vi "Goal Vision Align.vi"(10 "reinitialize? (F)":bool, 11 "Goal Vision Packet":T1) -> (1 "Heading Target":dbl, 2 "Aligned?":bool, 3 "Turn Power":dbl)   [LabVIEW 2015]
uses:
  Common Code/Goal Vision Packet.ctl
  Robot Global Data.vi
  <vilib>/addons/control/pid/pid.llb/PID (DBL).vi
  <vilib>/addons/control/pid/NI_PID_pid.lvlib
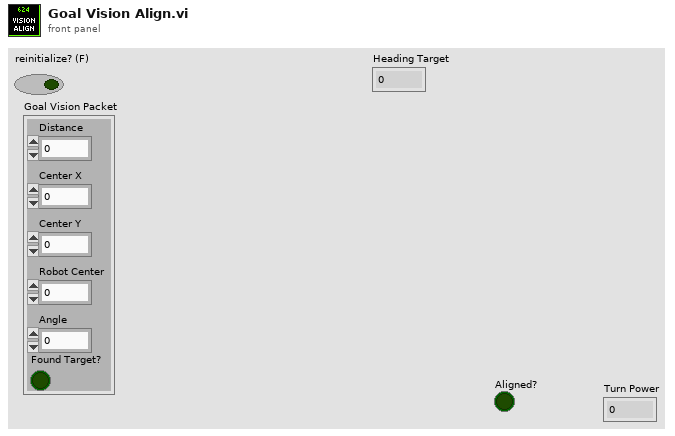
[diagram p1: front panel]
types:
  T1 = typedef "Goal Vision Packet.ctl" = cluster{"Distance":dbl, "Center X":dbl, "Center Y":dbl, "Found Target?":bool, "Robot Center":dbl, "Angle":dbl}
  T2 = typedef "Dashboard Control Data.ctl" = cluster{"Shooter Presets":T3, "Encoder Control":T5, "Steer PID output":cluster{"output high":dbl, "output low":dbl}, " Steer PID gains":cluster{"proportional gain (Kc)":dbl, "integral time (Ti, min)":dbl, "derivative time (Td, min)":dbl}, "Drivetrain Settings":T6, "Vision Packet":T1, "Dashboard Drivetrain Command":T7, "Info/Command Cluster":T9, "Ball Vision Packet":T10, "Intake Presets":T12, "Intake Encoder Control":T14, "Climb Presets":T15, "Goal Output Range":cluster{"output high":dbl, "output low":dbl}, "Enabled Systems":T16, "Auton Presets":T17, "Pressure M":dbl, "Pressure B":dbl}
  T3 = typedef "Shooter Presets.ctl" = cluster{"Batter Shot":T4, "Deep Middle":T4, "Manual Shot":T4, "Left Ticks Per Rotation":dbl, "Right Ticks Per Rotation":dbl, "Low Bar Shot":T4, "Shooter RPM Tolerance":dbl, "Trigger Power":dbl, "Fire from Load Delay":i32, "Max Angle":dbl, "Min Angle":dbl, "Angle PID gains":cluster{"P":dbl, "I":dbl, "D":dbl}, "Angle Output":cluster{"output high":dbl, "output low":dbl}, "Shooter Angle Tolerance":dbl, "Vision Shoot x^2":dbl, "Vision Shoot x":dbl, "Feed Forward Max Accel":dbl, "Feed Forward Kv":dbl, "Backwards Trigger":dbl, "Shot Finish Delay (ms)":dbl, "Angle Max Current":dbl, "Angle Current Trip Time":dbl, "Intake Angle":dbl, "Vision Shoot c":dbl, "Reset?":bool, "Button Release Delay":dbl, "Angle Pot x":dbl, "Angle Pot c":dbl, "Ignore Angle?":bool, "Max RPM":dbl, "Safty Frist Angle":dbl, "Intake Danger Height":dbl, "Angle Pot B":i32, "Angle Pot M":dbl, "FF Finish RPM":dbl, "RPM PID Right":cluster{"P":dbl, "I":dbl, "D":dbl, "FF":dbl}, "RPM PID Left":cluster{"P":dbl, "I":dbl, "D":dbl, "FF":dbl}, "Backwards RPM":dbl, "Vision RPM":dbl, "Run Wheels Backward Delay":u32, "Cleat Shot":T4}
  T4 = typedef "Shot Presets.ctl" = cluster{"L":dbl, "R":dbl, "A":dbl}
  T5 = typedef "Encoder Control.ctl" = cluster{"Right Tick Constant":dbl, "Left Tick Constant":dbl, "Reset?":bool, "Y Dist":cluster{"PID gains":cluster{"proportional gain (Kc)":dbl, "integral time (Ti, min)":dbl, "derivative time (Td, min)":dbl}}, "Y Stop Thresh":dbl, "Y Stop Speed":dbl}
  T6 = typedef "Drivetrain Settings.ctl" = cluster{"Gyro Tolerance":dbl, "Throttle Ramp (ms)":dbl, "Kv":dbl, "Ka":dbl, "Feed Forward P":dbl, "Feed Forward D":dbl, "Goal Vision PID gains":cluster{"proportional gain (Kc)":dbl, "integral time (Ti, min)":dbl, "derivative time (Td, min)":dbl}, "Goal Detection Window":dbl, "Creep Rate":dbl, "Vision Throttle Threshold":dbl, "Min Turn Output":dbl, "Left Batter Angle":dbl, "Right Batter Angle":dbl}
  T7 = typedef "Dashboard Drivetrain Command.ctl" = cluster{"Drivetrain Vision":T8}
  T8 = typedef "Drivetrain Vision.ctl" = cluster{"Goal Window":dbl, "Ball Window":dbl}
  T9 = typedef "Ball Tracking Command Cluster.ctl" = cluster{"Distance to Ball":dbl, "Desired Angle":dbl, "Command":enum16{"Turn to Ball", "Turn to Angle", "Get Distance"}, "Pixels from Center":dbl}
  T10 = typedef "Ball Vision Packet.ctl" = cluster{"Ball Detected?":bool, "Distance to Ball":dbl, "Desired Angle":dbl, "Pixels from Center":dbl, "Tracking mode":T11}
  T11 = typedef "Tracking Mode.ctl" = enum16{"Turn to Ball", "Turn to Angle"}
  T12 = typedef "Intake Presets.ctl" = cluster{"Intake Speed":dbl, "Outake Speed":dbl, "Low Height":dbl, "Half Height":dbl, "Full Height":dbl, "Angle Speed":dbl, "Angle Tolerance":dbl, "Encoder Scale":dbl, "Load Height":dbl, "Output Range":T13, "Rotation Power Max/Min":dbl, "MaxCurrent":dbl, "Intake Trip Time":dbl, "Idle Height":dbl, "Max Height":dbl, "Reset Encoders?":bool, "PID gains":cluster{"proportional gain (Kc)":dbl, "integral time (Ti, min)":dbl, "derivative time (Td, min)":dbl}, "Intake Stop Delay":u32, "Settle Time":dbl, "Settle Wait Time":dbl}
  T13 = typedef "Drivetrain Output Range.ctl" = cluster{"output high":dbl, "output low":dbl}
  T14 = typedef "IntakeEcoderControl.ctl" = cluster{"Arm Tick Constant":dbl, "Reset?":bool, "Y Dist":cluster{"PID gains":cluster{"proportional gain (Kc)":dbl, "integral time (Ti, min)":dbl, "derivative time (Td, min)":dbl}}, "Y Stop Thresh":dbl, "Y Stop Speed":dbl}
  T15 = typedef "Climb Presets.ctl" = cluster{"Pull Power":dbl, "Extend Power":dbl}
  T16 = typedef "Enabled Systems.ctl" = cluster{"Shoot":bool, "Intake":bool, "DT":bool, "Gyro":bool, "100ms":bool, "US":bool}
  T17 = typedef "Autonomous Presets.ctl" = cluster{"Pitch Limit":dbl, "Roll Limit":dbl, "Start Position":dbl, "Cross Position":dbl}
  T18 = cluster{"proportional gain (Kc)":dbl, "integral time (Ti, min)":dbl, "derivative time (Td, min)":dbl}
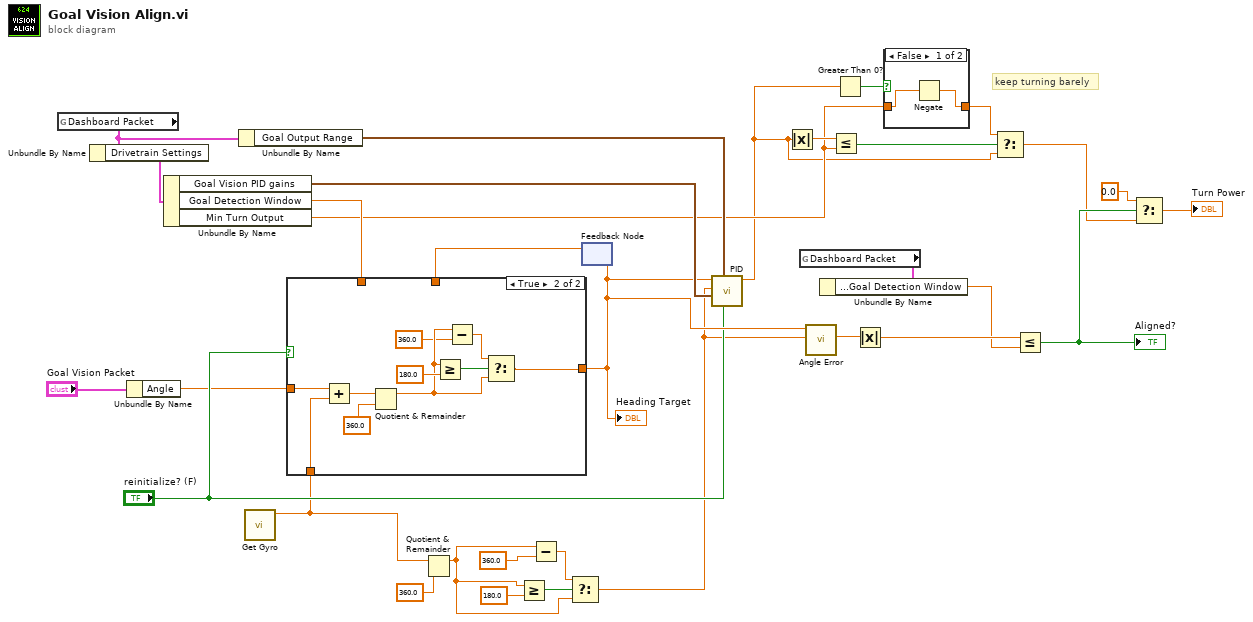
[diagram p0: block diagram]
diagram:
  # "keep turning barely"
  n1 = global read "Robot Global Data.vi" "Dashboard Packet"() -> (w27:T2)
  n2 = Unbundle By Name(w27) -> ("Drivetrain Settings"=w29:T6)
  n3 = Unbundle By Name("Goal Vision Packet") -> ("Angle"=w19:dbl)
  n4 = Unbundle By Name(w29) -> ("Goal Vision PID gains"=w31:T18, "Goal Detection Window"=w28:dbl, "Min Turn Output"=w7:dbl)
  n5 = Unbundle By Name(w27) -> ("Goal Output Range"=w30:cluster{"output high":dbl, "output low":dbl})
  n6 = call "Get Gyro.vi"() -> ("Angle"=w14:dbl)  [unwired: 11 in]
  n7 = Quotient & Remainder(x=w14, y=360.0) -> (x-y*floor(x/y)=w12:dbl)  [unwired: 1 out]
  n8 = Greater Or Equal?(x=w12, y=180.0) -> (x >= y?=w16:bool)
  n9 = Subtract(x=w12, y=360.0) -> (x-y=w18:dbl)
  n10 = Select(t=w18, s=w16, f=w12) -> (s? t:f=w11:dbl)
  n11 = feedback #1() -> (w26:dbl)  [unwired: 1 in]
  n12 = case shown="True" "reinitialize? (F)" {
    tunnel: w28 -> [_ _]
    tunnel: [w33 w34] -> w21
    tunnel: w14 -> [_ w43]
    tunnel: w26 -> [w33 _]
    tunnel: w19 -> [_ w40]
    frame False {
    }
    frame True {
      n13 = Add(x=w40, y=w43) -> (x+y=w41:dbl)
      n14 = Quotient & Remainder(x=w41, y=360.0) -> (x-y*floor(x/y)=w37:dbl)  [unwired: 1 out]
      n15 = Greater Or Equal?(x=w37, y=180.0) -> (x >= y?=w38:bool)
      n16 = Subtract(x=w37, y=360.0) -> (x-y=w35:dbl)
      n17 = Select(t=w35, s=w38, f=w37) -> (s? t:f=w34:dbl)
    }
  }
  "Heading Target" <- w21
  n18 = feedback-in #1(w21) -> ()
  n19 = call-poly <vilib>:"PID.vi"("reinitialize? (F)"="reinitialize? (F)", "output range"=w30, "PID gains"=w31, "process variable"=w11, "setpoint"=w21) -> ("output"=w5:dbl)  [unwired: 5 in, 1 out]
  n20 = Absolute Value(x=w5) -> (abs(x)=w10:dbl)
  n21 = global read "Robot Global Data.vi" "Dashboard Packet"() -> (w25:T2)
  n22 = call "Angle Error.vi"("Angle"=w11, "Target Angle"=w21) -> ("Error"=w24:dbl)  [unwired: 9 in]
  n23 = Unbundle By Name(w25) -> ("Drivetrain Settings.Goal Detection Window"=w22:dbl)
  n24 = Less Or Equal?(x=w10, y=w7) -> (x <= y?=w8:bool)
  n25 = Greater Than 0?(x=w5) -> (x > 0?=w9:bool)
  n26 = Absolute Value(x=w24) -> (abs(x)=w23:dbl)
  n27 = case shown="False" w9 {
    tunnel: w7 -> [w45 w46]
    tunnel: [w44 w46] -> w6
    frame False {
      n28 = Negate(x=w45) -> (-x=w44:dbl)
    }
    frame True {
    }
  }
  n29 = Select(t=w6, s=w8, f=w5) -> (s? t:f=w3:dbl)
  n30 = Less Or Equal?(x=w23, y=w22) -> (x <= y?=w4:bool)
  "Aligned?" <- w4
  n31 = Select(t=0.0, s=w4, f=w3) -> (s? t:f=→"Turn Power":dbl)
